vi "CDMA_TxMsgEncode.vi"(7 "ch_cap":dbl, 8 "error in (no error)":errorcluster caption="错误输入（无错误）", 9 "ch_bit_len":dbl, 10 "ch_char_msg":string, 11 "Path":path) -> (0 "error out":errorcluster caption="错误输出", 2 "pdch_data":dbl[](array[numeric]), 3 "Path Out":path)   [LabVIEW 2015]
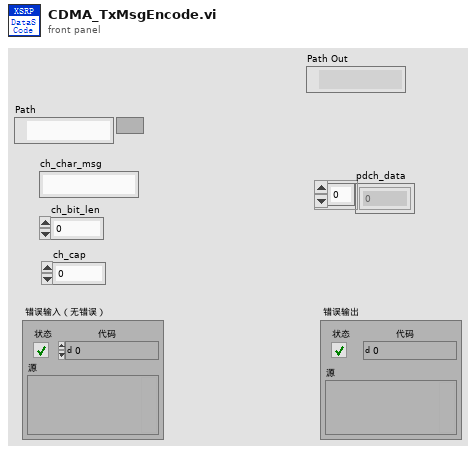
[diagram p1: front panel]
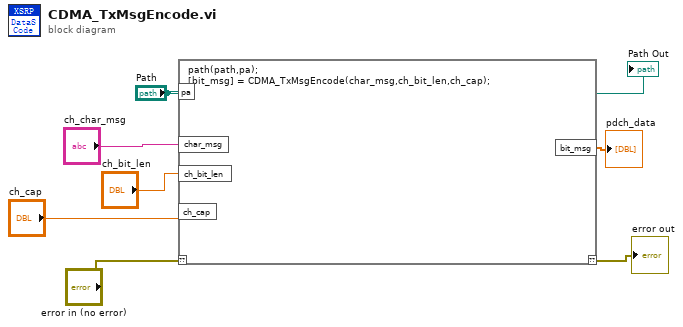
[diagram p0: block diagram]
diagram:
  n1 = script code="path(path,pa);\n[bit_msg] = CDMA_TxMsgEncode(char_msg,ch_bit_len,ch_cap);"("??"="error in (no error)", "pa"="Path", "char_msg"="ch_char_msg", "ch_bit_len"="ch_bit_len", "ch_cap"="ch_cap") -> ("??"=→"error out":errorcluster, "bit_msg"=→"pdch_data":dbl[])
  "Path Out" <- "Path"
